vi "createFilenameArray_slim.vi"(0 "no x steps":i32=1, 1 "no y steps":i32=1, 2 "no z steps":i32=1, 3 "No colours":i32=1, 4 "Base path":path=path "C:/Users/sims01/Desktop/dataAcq") -> (5 "stackFnameArray":path[][][](array[path]), 6 "frameFilenameArray":path[][][][](array[path]))   [LabVIEW 2015]
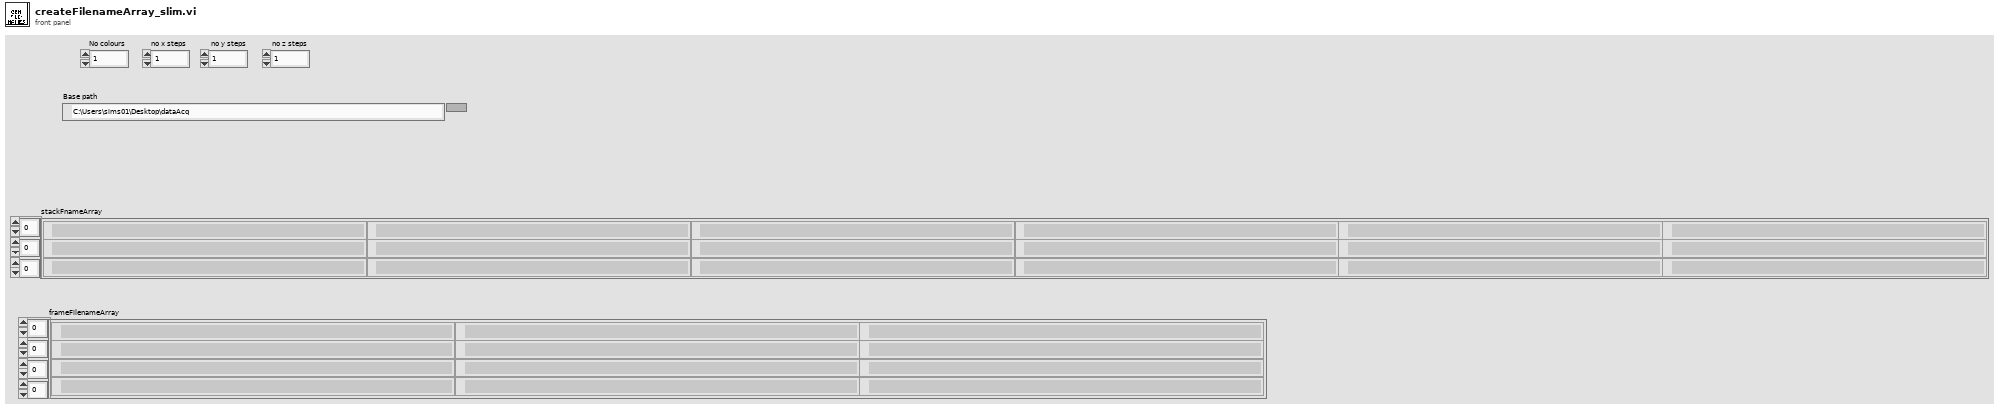
[diagram p1: front panel]
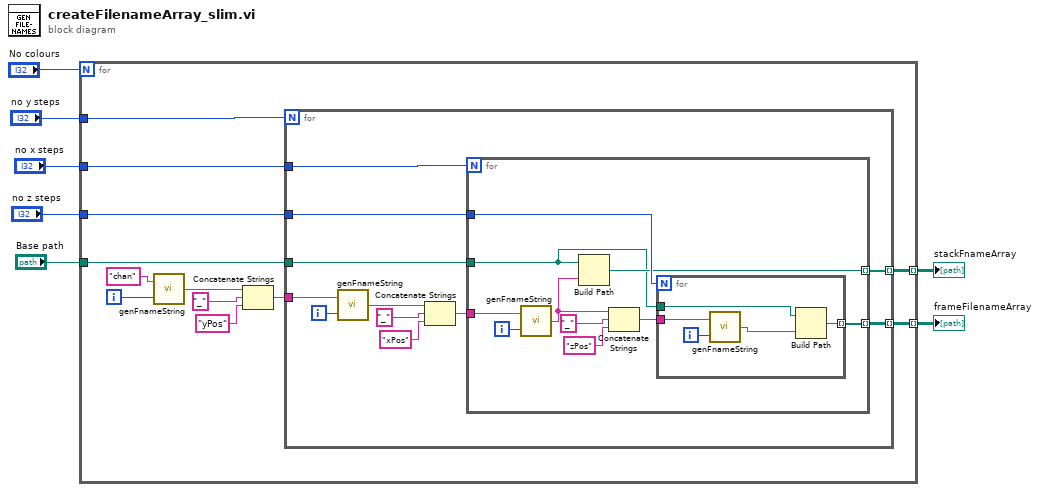
[diagram p0: block diagram]
diagram:
  n1 = for {
    N: "No colours" -> [_]
    tunnel: "no y steps" -> [w19]
    tunnel: "no x steps" -> [w18]
    tunnel: "no z steps" -> [w17]
    tunnel: [w14] -> w3 mode=indexing
    tunnel: "Base path" -> [w13]
    tunnel: [w12] -> w1 mode=indexing
    i -> [w16]
    n2 = call "genFnameString.vi"("Idx"=w16, "str"="chan") -> ("fName"=w10:string)
    n3 = Concatenate Strings(w10, "_" ("string"), "yPos") -> (w8:string)
    n4 = for {
      N: w19 -> [_]
      tunnel: w18 -> [w30]
      tunnel: w17 -> [w29]
      tunnel: [w27] -> w14 mode=indexing
      tunnel: w13 -> [w26]
      tunnel: [w25] -> w12 mode=indexing
      tunnel: w8 -> [w24]
      i -> [w28]
      n5 = call "genFnameString.vi"("Idx"=w28, "str"=w24) -> ("fName"=w23:string)
      n6 = Concatenate Strings(w23, "_" ("string"), "xPos") -> (w20:string)
      n7 = for {
        N: w30 -> [_]
        tunnel: w29 -> [w40]
        tunnel: [w38] -> w27 mode=indexing
        tunnel: w26 -> [w31]
        tunnel: [w37] -> w25 mode=indexing
        tunnel: w20 -> [w33]
        i -> [w39]
        n8 = call "genFnameString.vi"("Idx"=w39, "str"=w33) -> ("fName"=w32:string)
        n9 = Build Path(base path=w31, name or relative path=w32) -> (appended path=w37:path)
        n10 = Concatenate Strings(w32, "_" ("string"), "zPos") -> (w34:string)
        n11 = for {
          N: w40 -> [_]
          tunnel: [w44] -> w38 mode=indexing
          tunnel: w31 -> [w43]
          tunnel: w34 -> [w42]
          i -> [w45]
          n12 = call "genFnameString.vi"("Idx"=w45, "str"=w42) -> ("fName"=w41:string)
          n13 = Build Path(base path=w43, name or relative path=w41) -> (appended path=w44:path)
        }
      }
    }
  }
  "frameFilenameArray" <- w3
  "stackFnameArray" <- w1
